vi "Launch GUI.vi"(8 "error in":errorcluster, 11 "Series Actor in":refnum<class "Series Actor.lvclass">) -> (0 "error out":errorcluster, 3 "Series Actor out":refnum<class "Series Actor.lvclass">)   [LabVIEW 2024, in "Series Actor.lvlib" / "Series Actor.lvclass"]
uses:
  Series Actor.lvclass
  C:/Program Files/National Instruments/LabVIEW 2024/vi.lib/MGI/Panel Manager/Panel Actor/Panel Actor/Panel Actor.lvclass
  Series Actor.lvclass/Series Actor.ctl
  Series UI Actor/Series UI Actor/Series UI Actor.lvclass
  <vilib>/MGI/Panel Manager/Panel Actor/Panel Actor/Panel Actor.lvclass/Panel Actor.ctl
  9b8c0b92-681b-475e-8e76-d548d2c86d25.vi
  9b8c0b92-681b-475e-8e76-d548d2c86d25.vi/a4169a97-72fc-4003-a778-603cf20cafa0.vi
  <vilib>/JDP Science/JSONtext/Find Item.vi
  <vilib>/JDP Science/JSONtext/Next JSON Value.vi
  <vilib>/JDP Science/JSONtext/String Subset.vi
  <vilib>/JDP Science/JSONtext/Parsing/Advance past next JSON Value (inlined COPY).vi
  <vilib>/JDP Science/JSONtext/Parsing/Advance past whitespace.vi
  <vilib>/JDP Science/JSONtext/Parsing/Advance past String.vi
  <vilib>/JDP Science/JSONtext/Parsing/Advance past Number.vi
  <vilib>/JDP Science/JSONtext/Parsing/Advance past Line Ending.vi
  <vilib>/JDP Science/JSONtext/Parsing/Parse Full Path or Item Name.vi
  <vilib>/JDP Science/JSONtext/Parsing/Advance past Array.vi
  <vilib>/JDP Science/JSONtext/Parsing/Advance past Object.vi
  <vilib>/JDP Science/JSONtext/support/Error Cluster From Code.vi
  <vilib>/JDP Science/JSONtext/Offset/Find Item Locations by Path.vi
  <vilib>/JDP Science/JSONtext/JSON text to Variant.vi
  <vilib>/Utility/error.llb/Error Cluster From Error Code.vi
  <vilib>/JDP Science/JSONtext/LVClass Serializer/JSONtext LVClass Serializer.lvclass
  <vilib>/MGI/Panel Manager/Panel Actor/Panel Actor/Panel Actor.lvclass
  <vilib>/MGI/Panel Manager/Panel Actor/Panel Actor Messages/Show Panel Msg/Show Panel Msg.lvclass
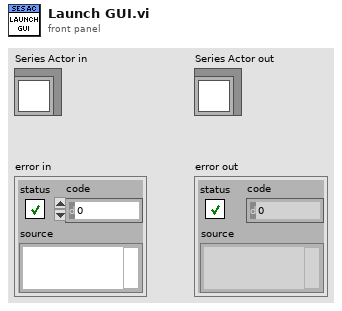
[diagram p1: front panel]
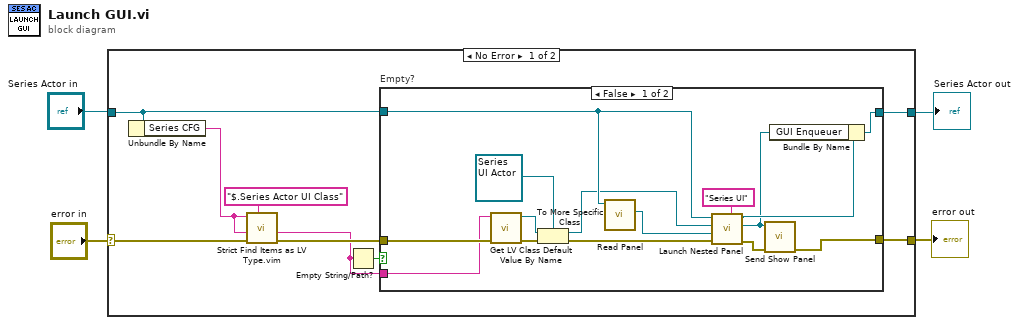
[diagram p0: block diagram]
diagram:
  n1 = case shown="No Error" "error in" {
    selector: "error in" -> [w13 w32]
    tunnel: [w10 w32] -> w2
    tunnel: [w11 w31] -> w1
    tunnel: "Series Actor in" -> [w7 w31]
    frame No Error {
      n2 = Unbundle By Name(w7) -> ("Series CFG"=w6:string)
      n3 = call "Strict Find Items as LV Type.vim"("$Path or Item Name"="$.Series Actor UI Class", "error in"=w13, "Data Type and Default Value"=w6, "<JSON>"=w6) -> ("error out"=w12:errorcluster, "Data out"=w5:string)  [unwired: 5 in, 1 out]
      n4 = Empty String/Path?(string/path=w5) -> (empty?=w8:bool)
      n5 = case "Empty?" shown="False" w8 {
        tunnel: w12 -> [w28 w30]
        tunnel: [w17 w29] -> w11
        tunnel: [w15 w30] -> w10
        tunnel: w5 -> [w25 _]
        tunnel: w7 -> [w20 w29]
        frame False {
          n6 = call <vilib>:"Get LV Class Default Value By Name.vi"("error in (no error)"=w28, "class name"=w25) -> ("error out"=w27:errorcluster, "object"=w26:refnum<class>)  [unwired: 8 in]
          n7 = To More Specific Class(target class=refnum<class "Series UI Actor.lvclass"> refnum ("Series UI Actor.lvlib:Series UI Actor.lvclass"), reference=w26, error in=w27) -> (specific class reference=w18:refnum<class "Series UI Actor.lvclass">, error out=w21:errorcluster)
          n8 = call <vilib>:"Read Panel.vi"("Panel Actor in"=w20) -> ("Panel"=w19:refnum<class "Panel.lvclass">)  [unwired: 10 in]
          n9 = call <vilib>:"Launch Nested Panel.vi"("Debug Alias"="Series UI", "error in (no error)"=w21, "Panel"=w19, "Nested Panel Actor"=w18, "Panel Actor in"=w20) -> ("error out"=w16:errorcluster, "Nested Actor's Enqueuer"=w14:refnum<class "Message Enqueuer.lvclass">, "Panel Actor out"=w23:refnum<class "Series Actor.lvclass">)  [unwired: 3 in, 1 out]
          n10 = call <vilib>:"Send Show Panel.vi"("Error In"=w16, "Message Enqueuer in"=w14) -> ("Error Out"=w15:errorcluster)  [unwired: 8 in, 1 out]
          n11 = Bundle By Name(cluster=w23, "GUI Enqueuer"=w14) -> (w17:refnum<class "Series Actor.lvclass">)
        }
        frame True {
        }
      }
    }
    frame Error {
    }
  }
  "error out" <- w2
  "Series Actor out" <- w1
